vi "探头模板-24-32-网络版.vi"(11 "探头序号":T11(ring) caption="探头地址") -> ()   [LabVIEW 2017]
panel:
  out "初始尺寸":T1
  out "定时循环结构名称":string="采集探头属性"
  in  "报警方式[]":string[](array[string])
  out "报警方式a":T2
  out "探头状态a":T3
  out "限值信息":string="<限值信息>"
  in  "探头属性":T4={"探头地址与信息"={"网络地址"="", "名称"="", "备注"="", "累积剂量"=0.0, "累积限值"=0.0, "硬件剂量率限值"=enum."一级限值", "剂量率限值1"=0.0, "剂量率限值2"=0.0, "报警方式"=enum."常报警"}, "测量值"={"时间"=timestamp(3554955153.6246996 s since 1904-01-01), "数值"=0.0}, "限值"={"限值1"=0.0, "限值2"=0.0, "探头限值"=enum."一级限值"}, "探头状态"=enum."正常", "累积记录"={"起始时间"=timestamp(0 s since 1904-01-01), "结束时间"=timestamp(0 s since 1904-01-01), "累积剂量"=0.0}, "报警方式"={"报警方式"=enum."常报警", "延迟计时"=0, "报警中？"=FALSE}}
  in  "停止":bool=TRUE
  out "探头地址":T11(ring)
  out "探头信息":string
  out "探头状态":enum16{"正常", "离线", "禁用", "一级报警", "二级报警", "累积报警"}(ring)=enum."禁用"
  out "测量值":dbl format="%.2g"
  out "单位":enum16{"μSv/h", "mSv/h"}(ring)
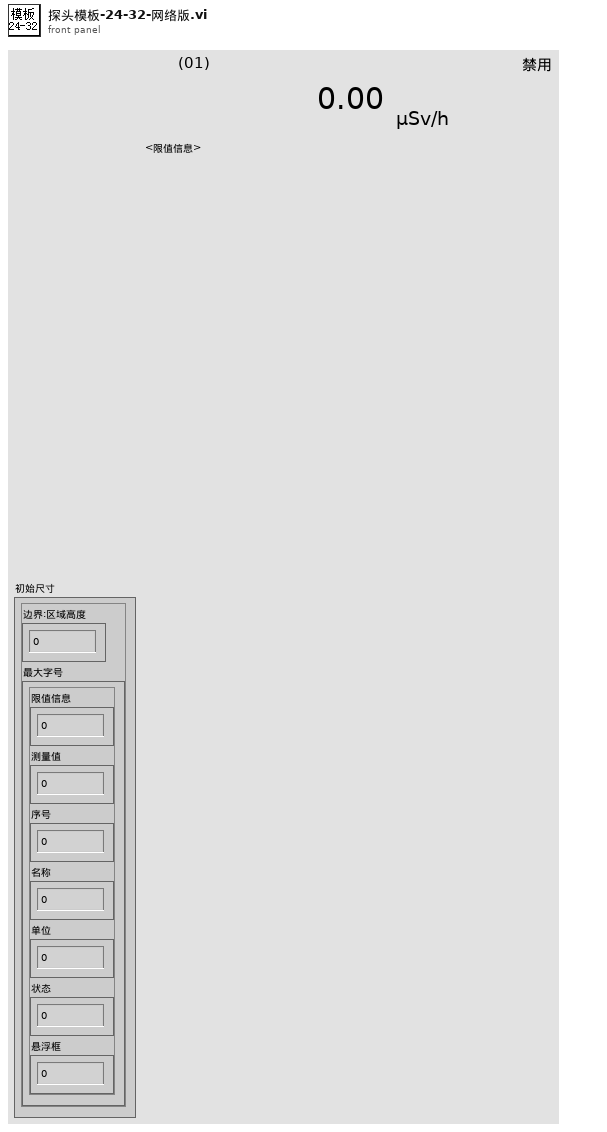
[diagram p1: front panel]
types:
  T1 = typedef "簇-界面模板初始字号.ctl" = cluster{"边界:区域高度":u32, "最大字号":cluster{"限值信息":u32, "测量值":u32, "序号":u32, "名称":u32, "单位":u32, "状态":u32, "悬浮框":u32}}
  T2 = typedef "报警方式选择.ctl" = enum16{"常报警", "自动静音", "手动静音"}
  T3 = typedef "探头状态.ctl" = enum16{"正常", "离线", "禁用", "一级报警", "二级报警", "累积报警"}
  T4 = typedef "探头属性.ctl" = cluster{"探头地址与信息":T5, "测量值":T7, "限值":T8, "探头状态":T3, "累积记录":T9, "报警方式":T10}
  T5 = typedef "探测器信息.ctl" = cluster{"网络地址":string, "名称":string, "备注":string, "累积剂量":dbl, "累积限值":dbl, "硬件剂量率限值":T6, "剂量率限值1":dbl, "剂量率限值2":dbl, "报警方式":T2}
  T6 = typedef "探头剂量率限值选择.ctl" = enum16{"一级限值", "二级限值"}
  T7 = typedef "测量值.ctl" = cluster{"时间":timestamp, "数值":dbl}
  T8 = typedef "剂量率限值.ctl" = cluster{"限值1":dbl, "限值2":dbl, "探头限值":T6}
  T9 = typedef "单条累积记录.ctl" = cluster{"起始时间":timestamp, "结束时间":timestamp, "累积剂量":dbl}
  T10 = typedef "报警方式.ctl" = cluster{"报警方式":T2, "延迟计时":u16, "报警中？":bool}
  T11 = enum16{"(01)", "(02)", "(03)", "(04)", "(05)", "(06)", "(07)", "(08)", "(09)", "(10)", "(11)", "(12)", "(13)", "(14)", "(15)", "(16)", "(17)", "(18)", "(19)", "(20)", "(21)", "(22)", "(23)", "(24)", "(25)", "(26)", "(27)", "(28)", "(29)", "(30)", "(31)", "(32)", "(33)", "(34)", "(35)"}
  T12 = cluster{"限值信息":u32, "测量值":u32, "序号":u32, "名称":u32, "单位":u32, "状态":u32, "悬浮框":u32}
  T13 = enum8{"Enabled", "Disabled", "Disabled and Grayed Out"}
  T14 = cluster{"原始尺寸":cluster{"所在窗格高度":u32, "字号":u32}, "new所在窗格高度":u32}
  T15 = enum16{"No Scaling", "Scale All Objects", "Scale Single Object"}
  T16 = typedef "LVRectTypeDef.ctl" = cluster{"Left":i16, "Top":i16, "Right":i16, "Bottom":i16}
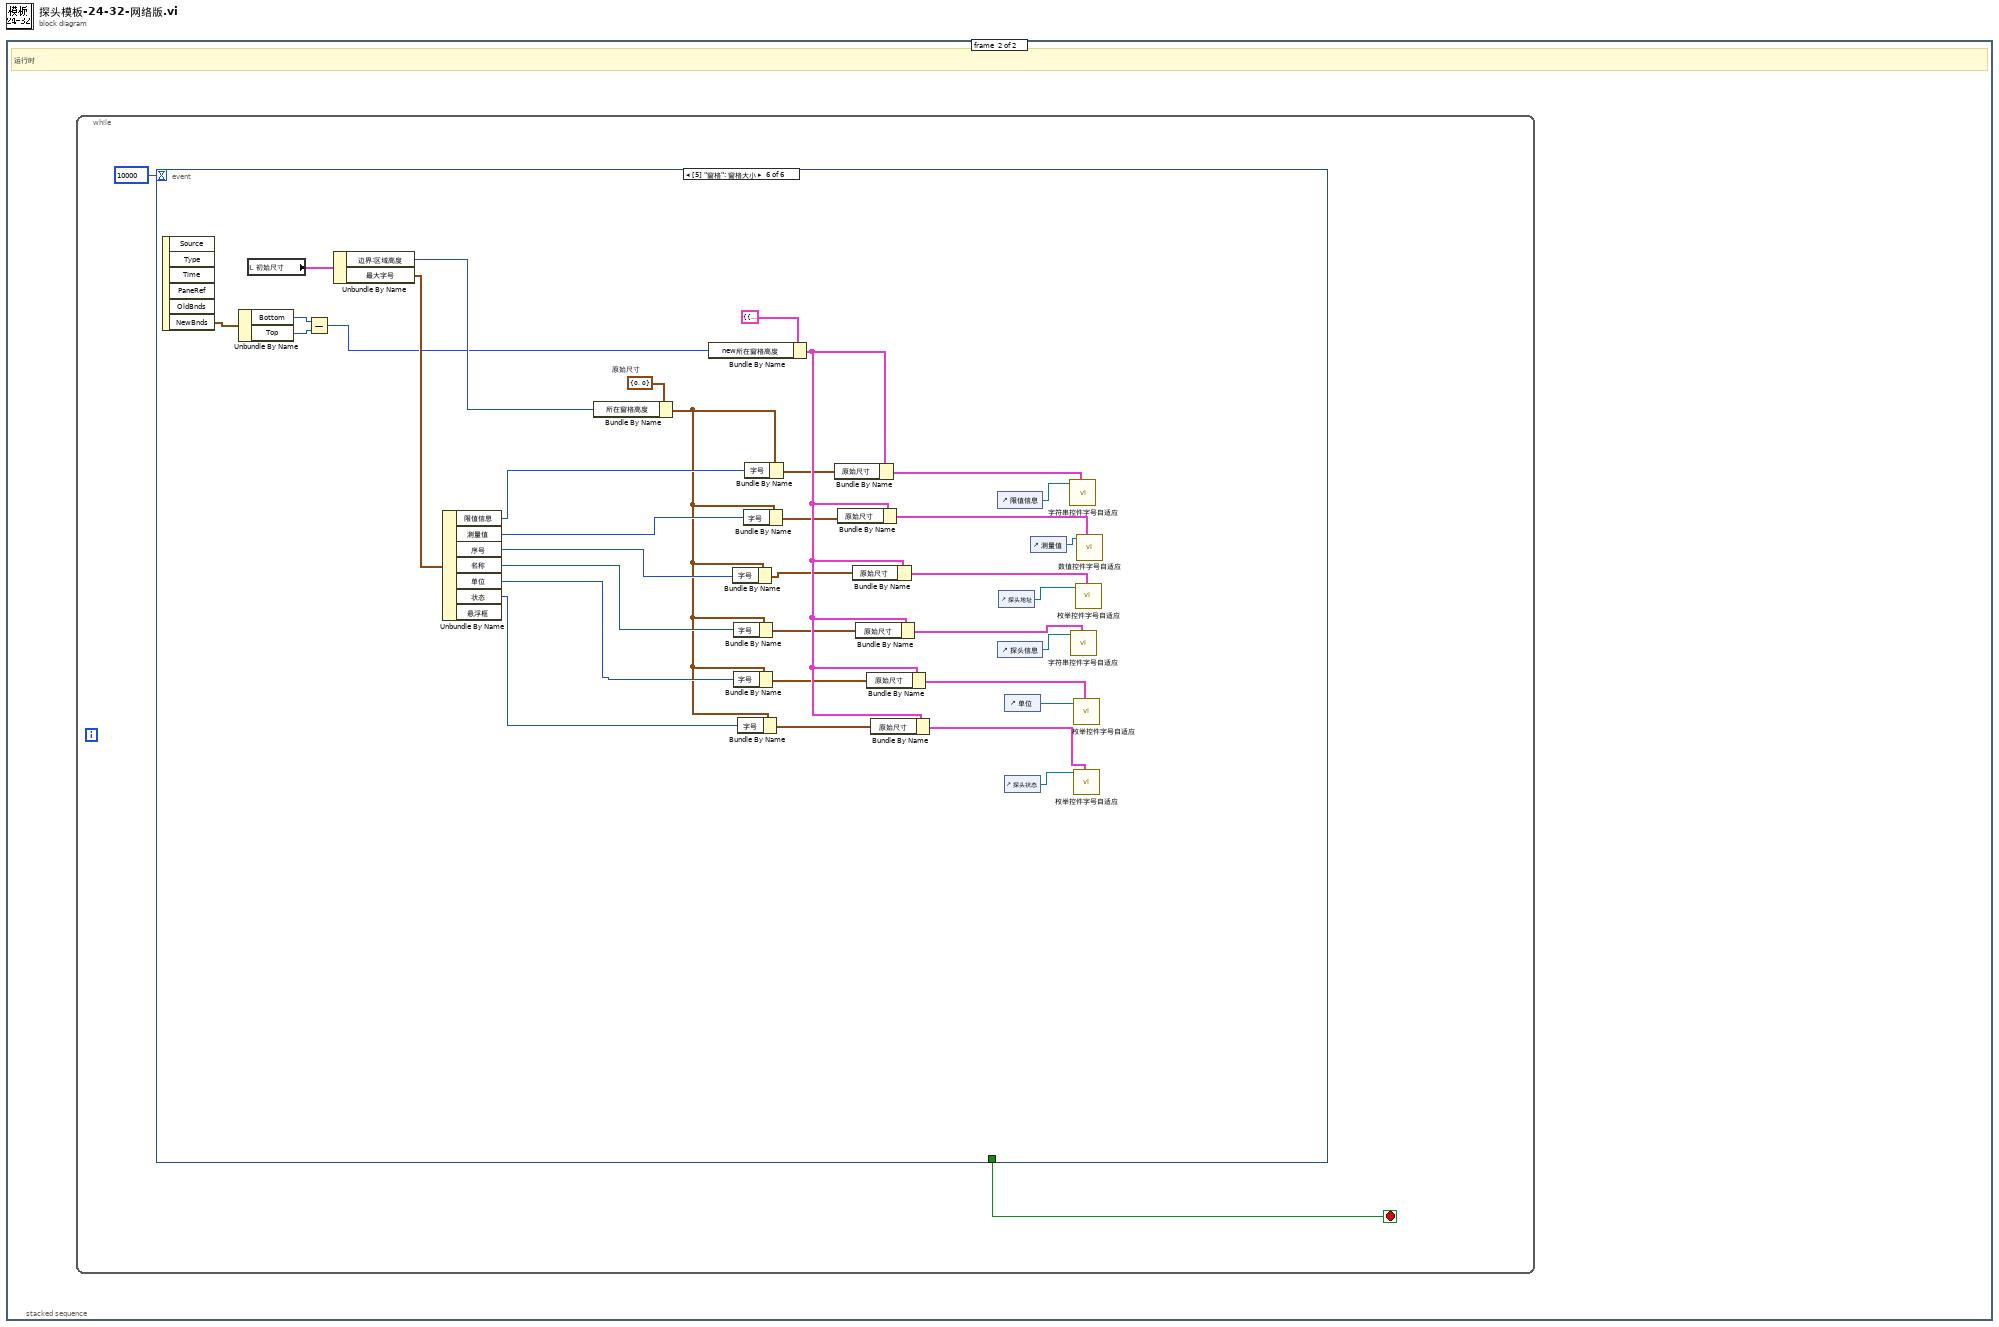
[diagram p0: block diagram]
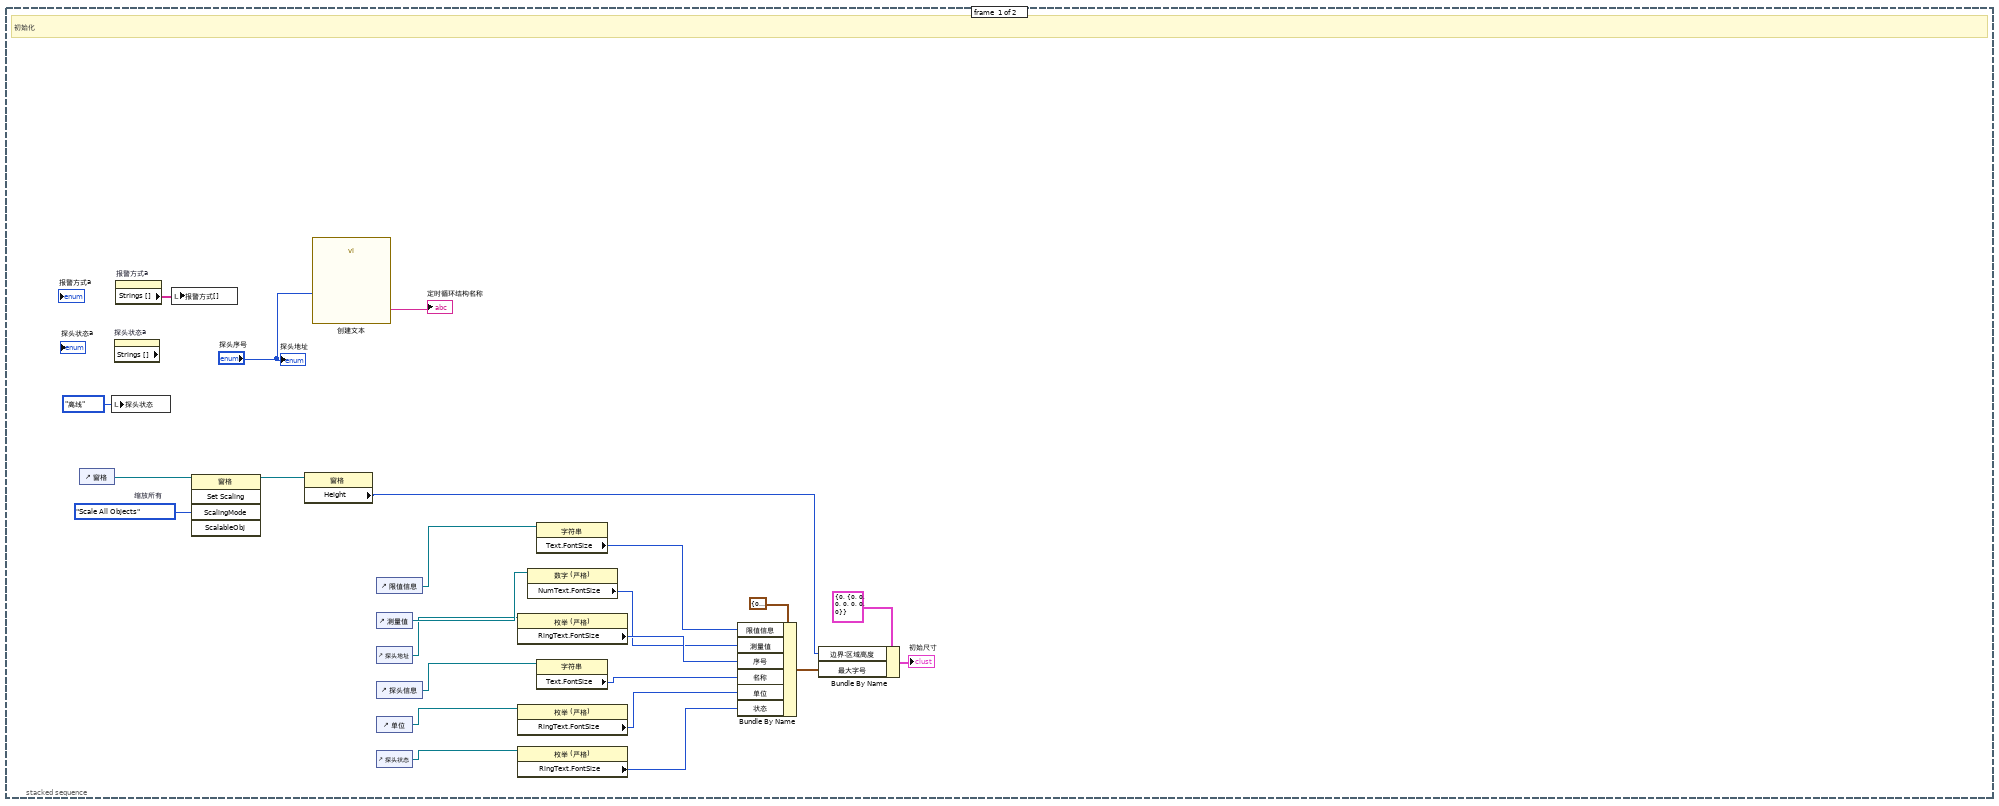
[diagram p2: hidden frame]
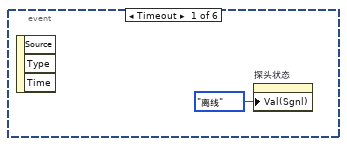
[diagram p3: hidden frame]
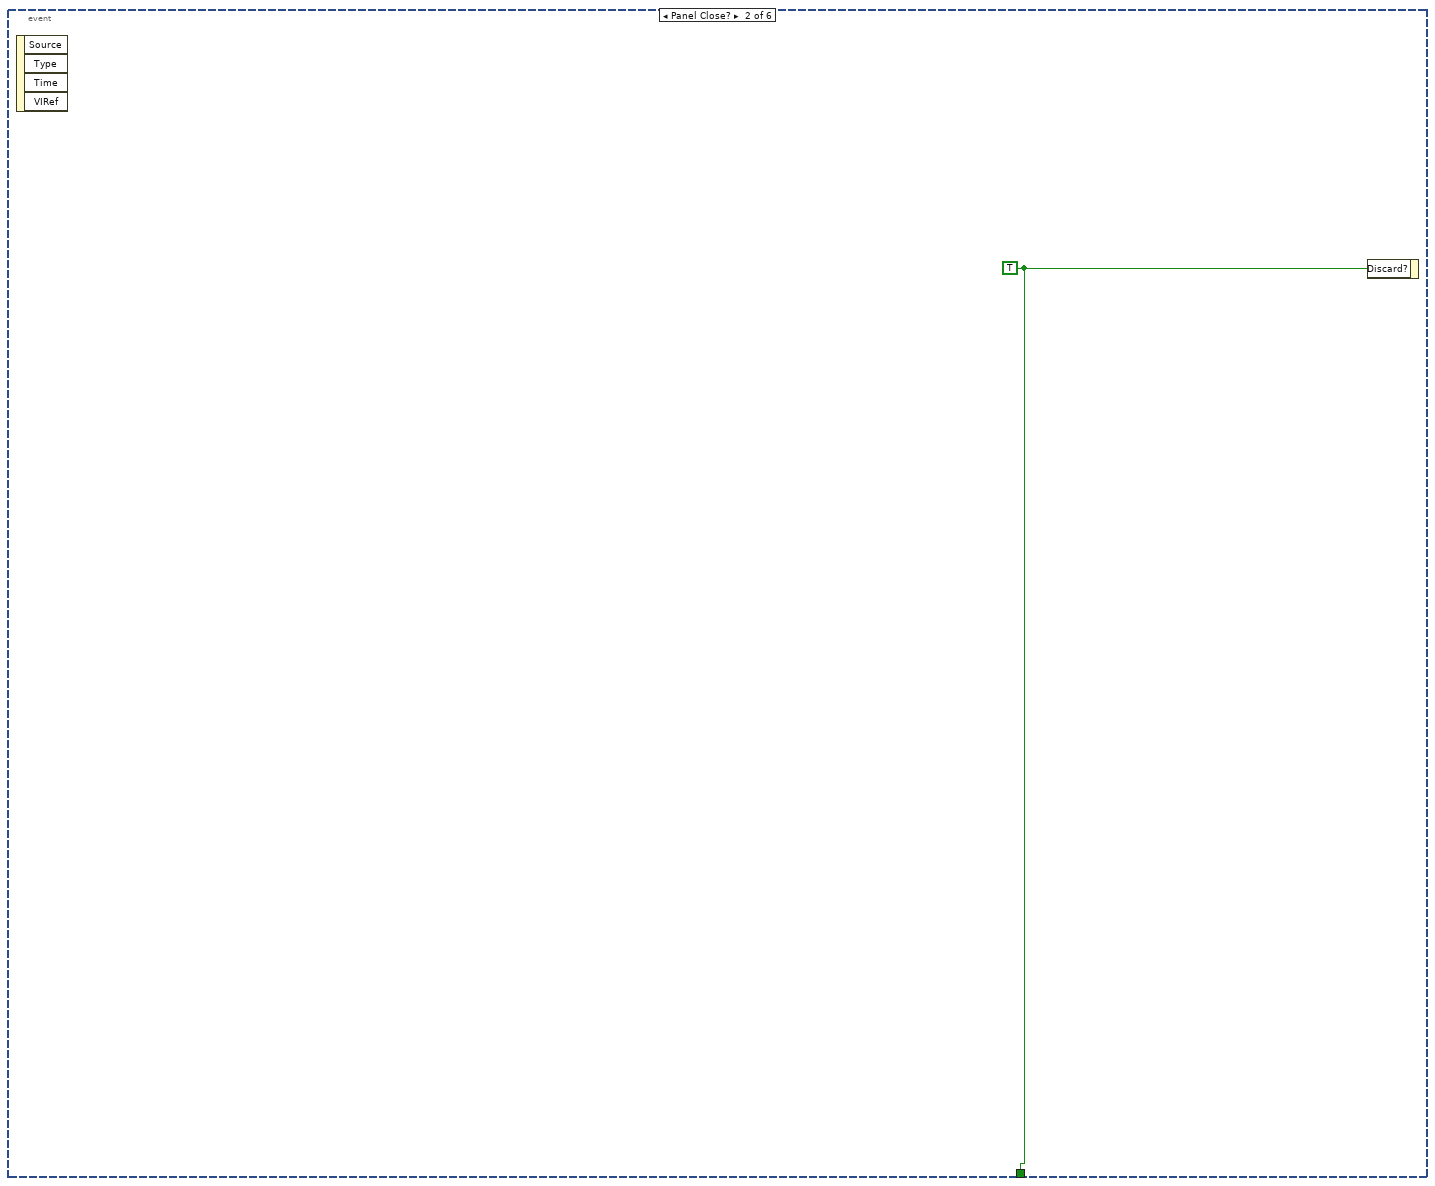
[diagram p4: hidden frame]
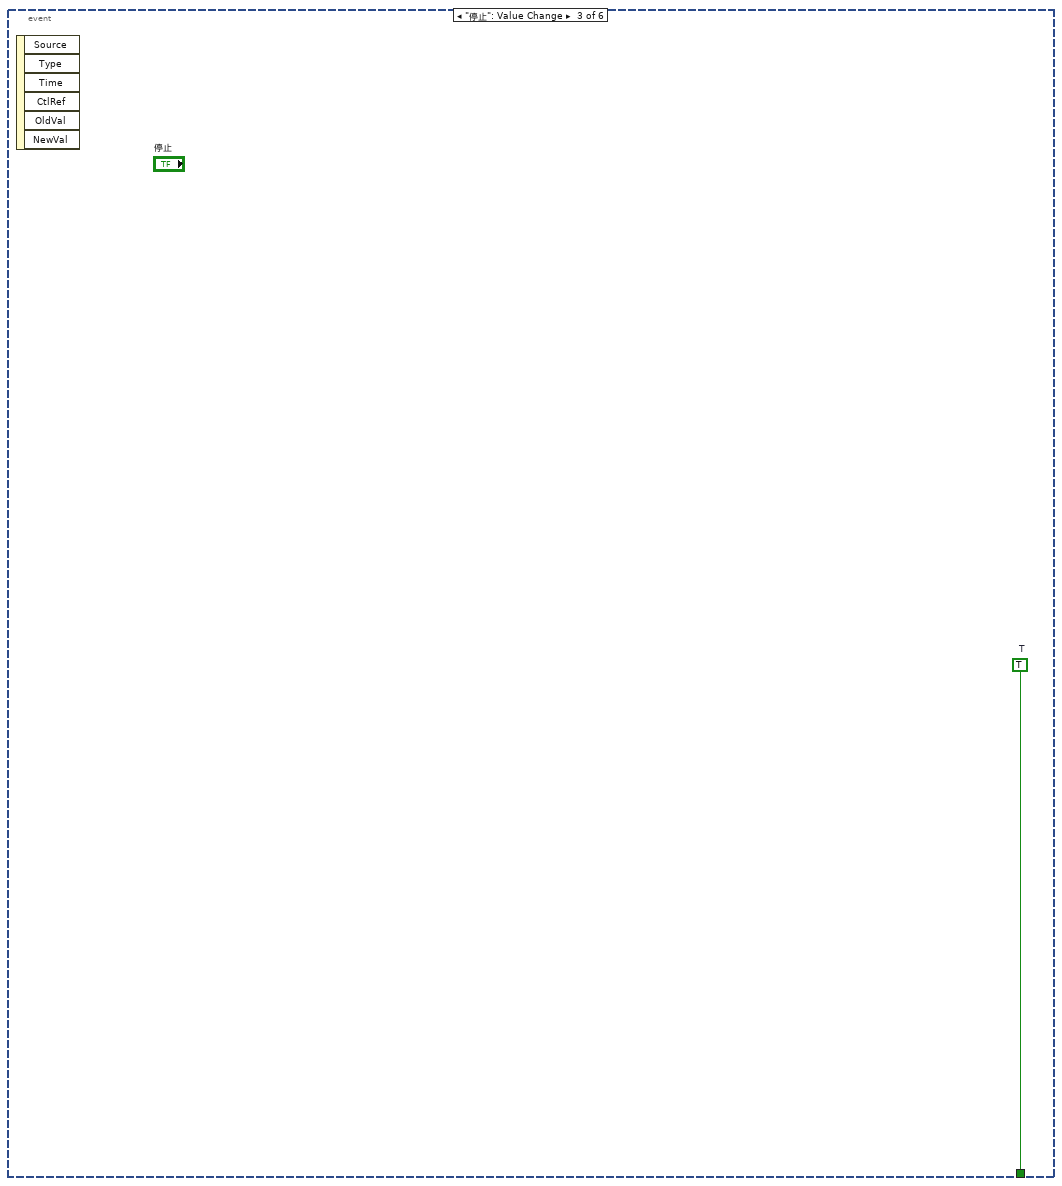
[diagram p5: hidden frame]
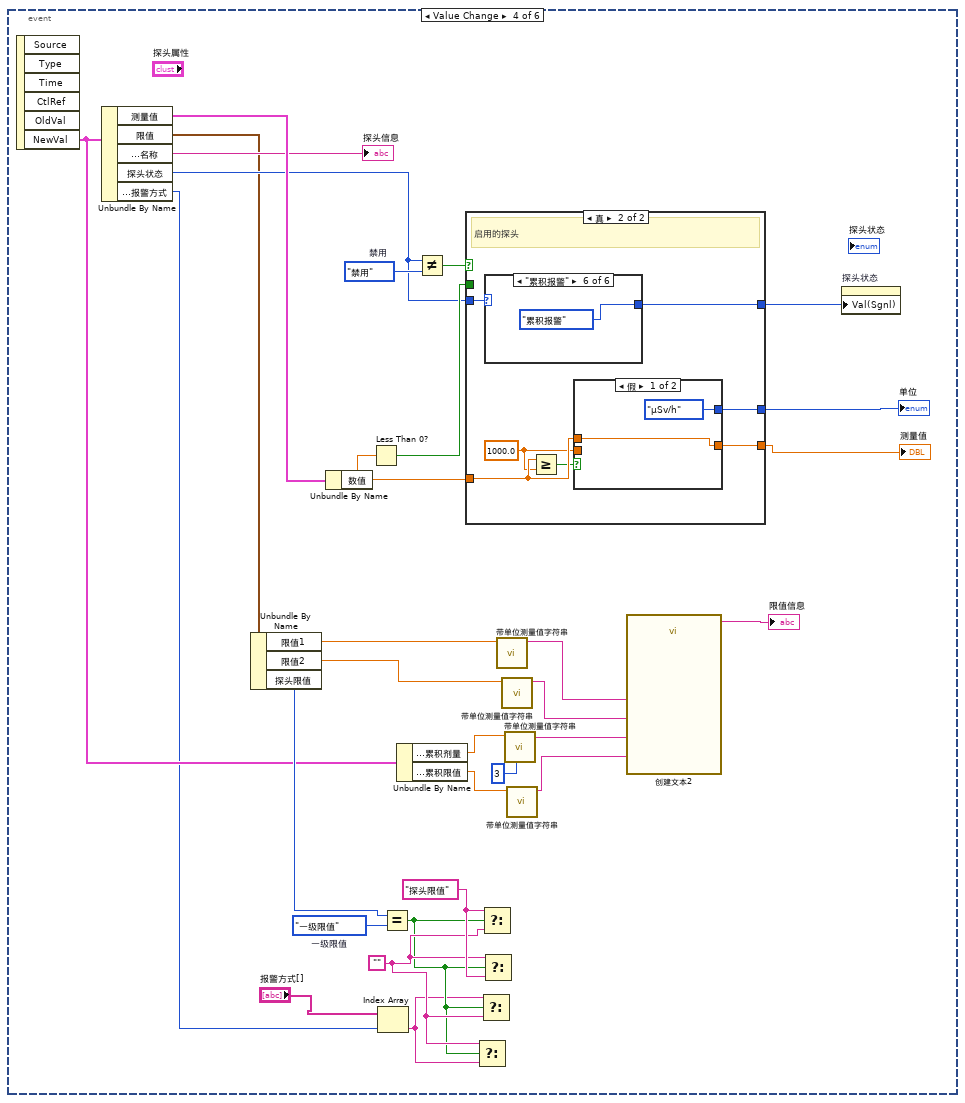
[diagram p6: hidden frame]
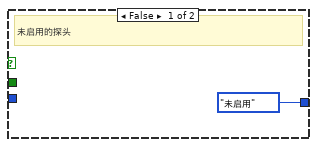
[diagram p7: hidden frame]
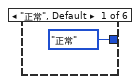
[diagram p8: hidden frame]
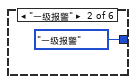
[diagram p9: hidden frame]
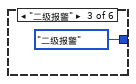
[diagram p10: hidden frame]
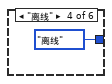
[diagram p11: hidden frame]
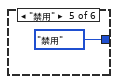
[diagram p12: hidden frame]
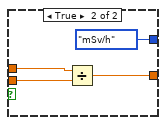
[diagram p13: hidden frame]
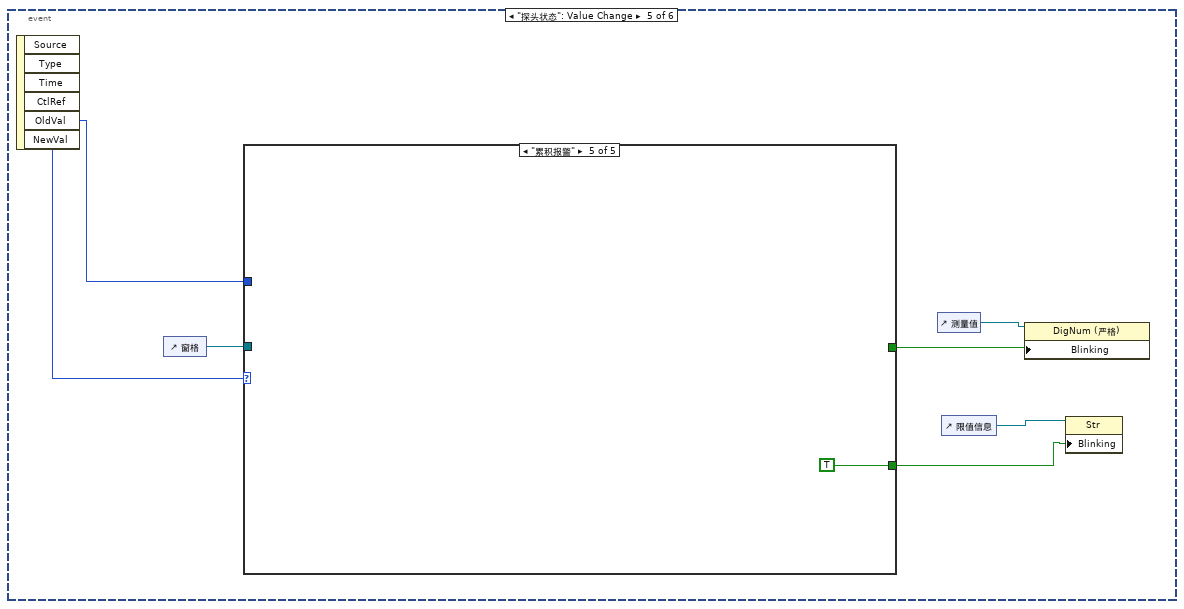
[diagram p14: hidden frame]
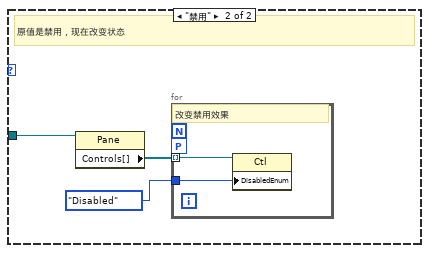
[diagram p16: hidden frame]
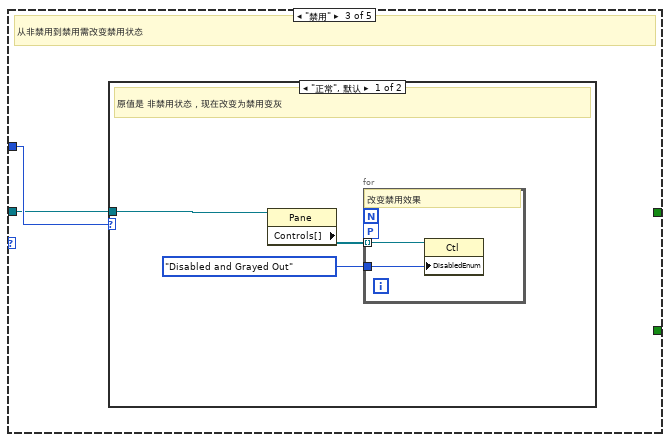
[diagram p18: hidden frame]
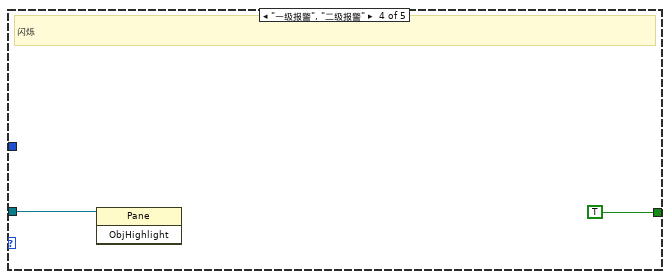
[diagram p20: hidden frame]
diagram:
  n1 = stacked-sequence {
    frame #0 {
      w19 = T15."Scale All Objects"  # 缩放所有
      # "初始化"
      n2 = control-ref of="窗格"() -> (w18:refnum<vi>)
      n3 = local write "探头状态"(探头状态."离线" ("探头状态")) -> ()
      n4 = property on="探头状态a" class="Enum (严格)" props=["Strings []"]() -> ()  [unwired: 2 in, 3 out]
      n5 = property on="报警方式a" class="Enum (严格)"() -> ("Strings []"=w23:string[])  [unwired: 2 in, 2 out]
      n6 = local write "报警方式[]"(w23) -> ()
      n7 = invoke class="窗格" method="Set Scaling"(reference=w18, "ScalingMode"=w19) -> (reference out=w20:refnum<vi>)  [unwired: 3 in, 4 out]
      n8 = property class="窗格"(reference=w20) -> ("Height"=w7:u32)  [unwired: 1 in, 2 out]
      n9 = call "创建文本"("序号"="探头序号") -> ("Result"=→"定时循环结构名称":string)  [unwired: 13 in, 1 out]
      n10 = control-ref of="限值信息"() -> (w6:refnum<vi>)
      n11 = control-ref of="测量值"() -> (w5:refnum<vi>)
      n12 = control-ref of="探头地址"() -> (w4:refnum<vi>)
      n13 = control-ref of="探头信息"() -> (w3:refnum<vi>)
      n14 = control-ref of="单位"() -> (w2:refnum<vi>)
      n15 = control-ref of="探头状态"() -> (w1:refnum<vi>)
      n16 = property class="枚举 (严格)"(reference=w4) -> ("RingText.FontSize"=w14:u32)  [unwired: 1 in, 2 out]
      n17 = property class="枚举 (严格)"(reference=w2) -> ("RingText.FontSize"=w16:u32)  [unwired: 1 in, 2 out]
      n18 = property class="枚举 (严格)"(reference=w1) -> ("RingText.FontSize"=w17:u32)  [unwired: 1 in, 2 out]
      n19 = property class="数字 (严格)"(reference=w5) -> ("NumText.FontSize"=w13:u32)  [unwired: 1 in, 2 out]
      n20 = property class="字符串"(reference=w6) -> ("Text.FontSize"=w12:u32)  [unwired: 1 in, 2 out]
      n21 = property class="字符串"(reference=w3) -> ("Text.FontSize"=w15:u32)  [unwired: 1 in, 2 out]
      n22 = Bundle By Name(cluster=T12 {"限值信息"=0, "测量值"=0, "序号"=0, "名称"=0, "单位"=0, "状态"=0, "悬浮框"=0} ("最大字号"), "限值信息"=w12, "测量值"=w13, "序号"=w14, "名称"=w15, "单位"=w16, "状态"=w17) -> (w8:T12)
      n23 = Bundle By Name(cluster=T1 {"边界:区域高度"=0, "最大字号"={"限值信息"=0, "测量值"=0, "序号"=0, "名称"=0, "单位"=0, "状态"=0, "悬浮框"=0}} ("输出簇"), "边界:区域高度"=w7, "最大字号"=w8) -> (→"初始尺寸":T1)
      "探头地址" <- "探头序号"
    }
    frame #1 {
      # "运行时"
      n24 = while {
        stop <- w25 stop-if-true
        n25 = event shown="[5] \"窗格\": 窗格大小" {
          selector: _ -> [_ _ _ _ _ _]
          dyn-events: _ -> [_ _ _ _ _ _]
          timeout: 10000 -> [_ _ _ _ _ _]
          tunnel: [_ w28 w29 _ _ _] -> w25
          event Timeout {
            n26 = event-data() -> ()  [unwired: 1 in, 3 out]
            n27 = property on="探头状态" class="Enum (严格)"("Val(Sgnl)"=探头状态."离线" ("值(信号)")) -> ()  [unwired: 2 in, 2 out]
          }
          event Panel Close? {
            w28 = TRUE ("放弃？")
            n28 = event-data() -> ()  [unwired: 1 in, 4 out]
            n29 = event-data("Discard?"=w28) -> ()  [unwired: 1 in, 1 out]
          }
          event "停止": Value Change {
            w29 = TRUE  # T
            n30 = event-data() -> ()  [unwired: 1 in, 6 out]
          }
          event Value Change {
            w46 = ""
            w47 = "探头限值" ("F-格式字符串")
            w48 = 探头剂量率限值选择."一级限值"  # 一级限值
            w52 = enum16{"正常", "离线", "禁用", "一级报警", "二级报警"}."禁用"  # 禁用
            n31 = event-data() -> ("NewVal"=w44:T4)  [unwired: 1 in, 5 out]
            n32 = Unbundle By Name(w44) -> ("测量值"=w54:T7, "限值"=w45:T8, "探头地址与信息.名称"=→"探头信息":string, "探头状态"=w50:T3, "探头地址与信息.报警方式"=w43:T2)
            n33 = Unbundle By Name(w45) -> ("限值1"=w38:dbl, "限值2"=w36:dbl, "探头限值"=w49:T6)
            n34 = Unbundle By Name(w54) -> ("数值"=w59:dbl)
            n35 = Less Than 0?(x=w59) -> (x < 0?=w58:bool)
            n36 = Index Array(array="报警方式[]", index=w43) -> (element=w41:string)
            n37 = Equal?(x=w49, y=w48) -> (x = y?=w42:bool)
            n38 = Unbundle By Name(w44) -> ("探头地址与信息.累积剂量"=w34:dbl, "探头地址与信息.累积限值"=w35:dbl)
            n39 = Not Equal?(x=w50, y=w52) -> (x != y?=w51:bool)
            n40 = case shown="真" w51 {
              tunnel: w58 -> [_ _]
              tunnel: w59 -> [_ w67]
              tunnel: [_ w66] -> w56
              tunnel: [_ w65] -> w57
              tunnel: [enum16{"正常", "未启用", "离线", "一级报警", "二级报警"}."未启用" ("探头状态") w64] -> w55
              tunnel: w50 -> [_ w63]
              frame False {
                # "未启用的探头"
              }
              frame True {
                w61 = 1000.0 ("y")
                # "启用的探头"
                n41 = case shown="\"累积报警\"" w63 {
                  tunnel: [探头状态."正常" ("探头状态") 探头状态."一级报警" ("探头状态") 探头状态."二级报警" ("探头状态") 探头状态."离线" ("探头状态") 探头状态."禁用" ("探头状态") 探头状态."累积报警" ("探头状态")] -> w64
                  frame "正常", Default {
                  }
                  frame "一级报警" {
                  }
                  frame "二级报警" {
                  }
                  frame "离线" {
                  }
                  frame "禁用" {
                  }
                  frame "累积报警" {
                  }
                }
                n42 = Greater Or Equal?(x=w67, y=w61) -> (x >= y?=w62:bool)
                n43 = case shown="假" w62 {
                  tunnel: w67 -> [w75 w79]
                  tunnel: w61 -> [_ w78]
                  tunnel: [w75 w77] -> w66
                  tunnel: [enum16{"μSv/h", "mSv/h"}."μSv/h" ("单位") enum16{"μSv/h", "mSv/h"}."mSv/h" ("单位")] -> w65
                  frame False {
                  }
                  frame True {
                    n44 = Divide(x=w79, y=w78) -> (x/y=w77:dbl)
                  }
                }
              }
            }
            "测量值" <- w56
            "单位" <- w57
            n45 = Select(t=w46, s=w42, f=w41) -> ()  [unwired: 1 out]
            n46 = Select(t=w41, s=w42, f=w46) -> ()  [unwired: 1 out]
            n47 = Select(t=w47, s=w42, f=w46) -> ()  [unwired: 1 out]
            n48 = Select(t=w46, s=w42, f=w47) -> ()  [unwired: 1 out]
            n49 = call "带单位测量值字符串.vi"("测量值"=w38) -> ("结果"=w37:string)  [unwired: 10 in]
            n50 = call "带单位测量值字符串.vi"("测量值"=w36) -> ("结果"=w30:string)  [unwired: 10 in]
            n51 = call "带单位测量值字符串.vi"("精度(2)"=i16 3 ("精度(6)"), "测量值"=w34) -> ("结果"=w33:string)  [unwired: 9 in]
            n52 = call "带单位测量值字符串.vi"("测量值"=w35) -> ("结果"=w32:string)  [unwired: 10 in]
            n53 = call "创建文本2"("累积限值"=w32, "一级"=w37, "二级"=w30, "累积"=w33) -> ("Result"=→"限值信息":string)  [unwired: 10 in, 1 out]
            n54 = property on="探头状态" class="Enum (严格)"("Val(Sgnl)"=w55) -> ()  [unwired: 2 in, 2 out]
          }
          event "探头状态": Value Change {
            n55 = event-data() -> ("OldVal"=w85:enum16{"正常", "离线", "禁用", "一级报警", "二级报警", "累积报警"}, "NewVal"=w84:enum16{"正常", "离线", "禁用", "一级报警", "二级报警", "累积报警"})  [unwired: 1 in, 4 out]
            n56 = control-ref of="窗格"() -> (w86:refnum<vi>)
            n57 = case shown="\"累积报警\"" w84 {
              tunnel: w85 -> [w88 _ w95 _ _]
              tunnel: w86 -> [w87 _ w94 w102 _]
              tunnel: [_ _ _ _ TRUE] -> w81
              tunnel: [_ _ _ TRUE _] -> w80
              frame "正常", Default {
                # "从禁用到正常 需改变禁用状态"
                n58 = case shown="\"正常\", 默认" w88 {
                  tunnel: w87 -> [_ w90]
                  frame "正常", Default {
                  }
                  frame "禁用" {
                    # "原值是禁用，现在改变状态"
                    n59 = property class="Pane"(reference=w90) -> ("Controls[]"=w91:refnum<vi>[])  [unwired: 1 in, 2 out]
                    n60 = for {
                      tunnel: w91 -> [w93] mode=indexing
                      workers-P: _ -> [_]
                      tunnel: T13."Disabled" ("禁用") -> [w92]
                      # "改变禁用效果"
                      n61 = property class="Ctl"(reference=w93, "DisabledEnum"=w92) -> ()  [unwired: 1 in, 2 out]
                    }
                  }
                }
              }
              frame "离线" {
                # "无需动作"
              }
              frame "禁用" {
                # "从非禁用到禁用需改变禁用状态"
                n62 = case shown="\"正常\", 默认" w95 {
                  tunnel: w94 -> [w97 _]
                  frame "正常", Default {
                    # "原值是 非禁用状态，现在改变为禁用变灰"
                    n63 = property class="Pane"(reference=w97) -> ("Controls[]"=w98:refnum<vi>[])  [unwired: 1 in, 2 out]
                    n64 = for {
                      tunnel: w98 -> [w100] mode=indexing
                      workers-P: _ -> [_]
                      tunnel: T13."Disabled and Grayed Out" ("禁用") -> [w99]
                      # "改变禁用效果"
                      n65 = property class="Ctl"(reference=w100, "DisabledEnum"=w99) -> ()  [unwired: 1 in, 2 out]
                    }
                  }
                  frame "禁用" {
                    # "原来就是禁用状态，不改变"
                  }
                }
              }
              frame "一级报警", "二级报警" {
                # "闪烁"
                n66 = invoke class="Pane" method="ObjHighlight"(reference=w102) -> ()  [unwired: 2 in, 3 out]
              }
              frame "累积报警" {
              }
            }
            n67 = control-ref of="测量值"() -> (w83:refnum<vi>)
            n68 = control-ref of="限值信息"() -> (w82:refnum<vi>)
            n69 = property class="DigNum (严格)"(reference=w83, "Blinking"=w80) -> ()  [unwired: 1 in, 2 out]
            n70 = property class="Str"(reference=w82, "Blinking"=w81) -> ()  [unwired: 1 in, 2 out]
          }
          event Pane Size {
            w120 = cluster{"所在窗格高度":u32, "字号":u32} {"所在窗格高度"=0, "字号"=0}  # 原始尺寸
            n71 = event-data() -> ("NewBnds"=w130:T16)  [unwired: 1 in, 5 out]
            n72 = Unbundle By Name(w130) -> ("Bottom"=w132:i16, "Top"=w131:i16)
            n73 = local read "初始尺寸"() -> (w112:T1)
            n74 = Subtract(x=w132, y=w131) -> (x-y=w111:i16)
            n75 = Unbundle By Name(w112) -> ("边界:区域高度"=w122:u32, "最大字号"=w113:T12)
            n76 = Unbundle By Name(w113) -> ("限值信息"=w123:u32, "测量值"=w124:u32, "序号"=w125:u32, "名称"=w126:u32, "单位"=w127:u32, "状态"=w128:u32)  [unwired: 1 out]
            n77 = Bundle By Name(cluster=w120, "所在窗格高度"=w122) -> (w106:cluster{"所在窗格高度":u32, "字号":u32})
            n78 = Bundle By Name(cluster=T14 {"原始尺寸"={"所在窗格高度"=0, "字号"=0}, "new所在窗格高度"=0} ("输出簇"), "new所在窗格高度"=w111) -> (w129:T14)
            n79 = Bundle By Name(cluster=w106, "字号"=w125) -> (w117:cluster{"所在窗格高度":u32, "字号":u32})
            n80 = Bundle By Name(cluster=w106, "字号"=w126) -> (w116:cluster{"所在窗格高度":u32, "字号":u32})
            n81 = Bundle By Name(cluster=w106, "字号"=w127) -> (w115:cluster{"所在窗格高度":u32, "字号":u32})
            n82 = Bundle By Name(cluster=w106, "字号"=w128) -> (w114:cluster{"所在窗格高度":u32, "字号":u32})
            n83 = Bundle By Name(cluster=w106, "字号"=w124) -> (w118:cluster{"所在窗格高度":u32, "字号":u32})
            n84 = Bundle By Name(cluster=w106, "字号"=w123) -> (w119:cluster{"所在窗格高度":u32, "字号":u32})
            n85 = Bundle By Name(cluster=w129, "原始尺寸"=w119) -> (w110:T14)
            n86 = Bundle By Name(cluster=w129, "原始尺寸"=w118) -> (w109:T14)
            n87 = Bundle By Name(cluster=w129, "原始尺寸"=w117) -> (w108:T14)
            n88 = Bundle By Name(cluster=w129, "原始尺寸"=w116) -> (w107:T14)
            n89 = Bundle By Name(cluster=w129, "原始尺寸"=w115) -> (w105:T14)
            n90 = Bundle By Name(cluster=w129, "原始尺寸"=w114) -> (w104:T14)
            n91 = control-ref of="限值信息"() -> (w137:refnum<vi>)
            n92 = control-ref of="探头信息"() -> (w138:refnum<vi>)
            n93 = control-ref of="探头地址"() -> (w134:refnum<vi>)
            n94 = control-ref of="单位"() -> (w135:refnum<vi>)
            n95 = control-ref of="探头状态"() -> (w136:refnum<vi>)
            n96 = control-ref of="测量值"() -> (w133:refnum<vi>)
            n97 = call "字符串控件字号自适应.vi"("新旧尺寸信息"=w110, "字符串控件-引用"=w137) -> ()  [unwired: 8 in, 2 out]
            n98 = call "字符串控件字号自适应.vi"("新旧尺寸信息"=w107, "字符串控件-引用"=w138) -> ()  [unwired: 8 in, 2 out]
            n99 = call "枚举控件字号自适应.vi"("新旧尺寸信息"=w105, "枚举控件-引用"=w135) -> ()  [unwired: 8 in, 2 out]
            n100 = call "枚举控件字号自适应.vi"("新旧尺寸信息"=w104, "枚举控件-引用"=w136) -> ()  [unwired: 8 in, 2 out]
            n101 = call "枚举控件字号自适应.vi"("新旧尺寸信息"=w108, "枚举控件-引用"=w134) -> ()  [unwired: 8 in, 2 out]
            n102 = call "数值控件字号自适应.vi"("新旧尺寸信息"=w109, "数值控件-引用"=w133) -> ()  [unwired: 8 in, 2 out]
          }
        }
      }
    }
  }
